vi "Update Histogram Window Menu Checks.vi"(8 "Error In":errorcluster, 9 "menu reference":refnum<k9>, 11 "XYGraph in":refnum<vi>) -> (0 "Error Out":errorcluster)   [LabVIEW 2019, in "Histogram Window.lvlib"]
uses:
  Histogram Window.lvlib
  Graphs/XY Graph/XY Graph Add-Ons.lvlib
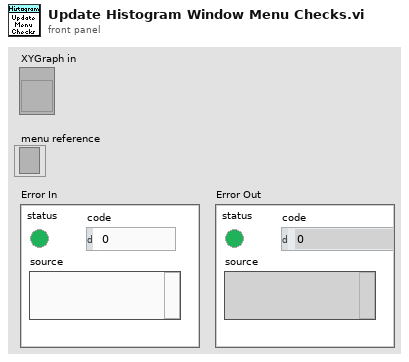
[diagram p1: front panel]
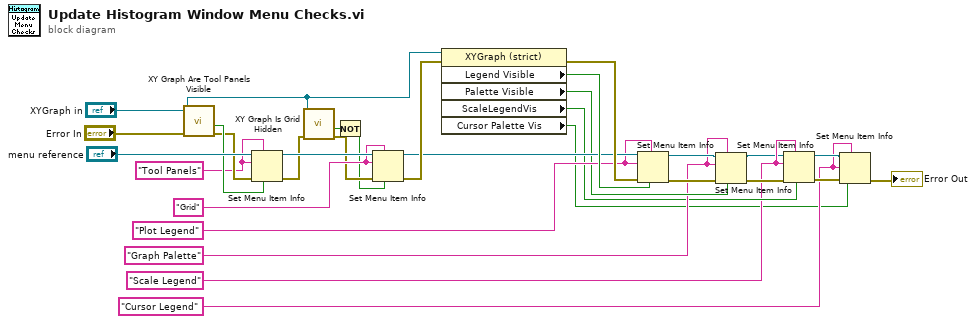
[diagram p0: block diagram]
diagram:
  w24 = "Grid" ("item name")
  w8 = "Cursor Legend" ("item name")
  w12 = "Scale Legend" ("item name")
  w15 = "Graph Palette" ("item name")
  w19 = "Plot Legend" ("item name")
  w27 = "Tool Panels" ("item name")
  n1 = call "XY Graph Are Tool Panels Visible.vi"("Error In"="Error In", "XY Graph Ref"="XYGraph in") -> ("Error Out"=w28:errorcluster, "Any Panel Visible?"=w29:bool)  [unwired: 7 in, 1 out]
  n2 = Set Menu Item Info(6:w29, 7:w27, 8:w28, 10:w27, 11:"menu reference") -> (0:w5:errorcluster, 3:w25:refnum<k9>)  [unwired: 2 in]
  n3 = call "XY Graph Is Grid Hidden.vi"("Error In"=w5, "XY Graph Ref"="XYGraph in") -> ("Error Out (dup)"=w4:errorcluster, "Hidden Grid(s)"=w3:bool)  [unwired: 7 in, 1 out]
  n4 = Not(x=w3) -> (.not. x?=w2:bool)
  n5 = Set Menu Item Info(6:w2, 7:w24, 8:w4, 10:w24, 11:w25) -> (0:w23:errorcluster, 3:w20:refnum<k9>)  [unwired: 2 in]
  n6 = property class="XYGraph (strict)"(reference="XYGraph in", error in=w23) -> (error out=w21:errorcluster, "Legend Visible"=w22:bool, "Palette Visible"=w16:bool, "ScaleLegendVis"=w13:bool, "Cursor Palette Vis"=w7:bool)  [unwired: 1 out]
  n7 = Set Menu Item Info(6:w22, 7:w19, 8:w21, 10:w19, 11:w20) -> (0:w18:errorcluster, 3:w17:refnum<k9>)  [unwired: 2 in]
  n8 = Set Menu Item Info(6:w16, 7:w15, 8:w18, 10:w15, 11:w17) -> (0:w14:errorcluster, 3:w9:refnum<k9>)  [unwired: 2 in]
  n9 = Set Menu Item Info(6:w13, 7:w12, 8:w14, 10:w12, 11:w9) -> (0:w11:errorcluster, 3:w10:refnum<k9>)  [unwired: 2 in]
  n10 = Set Menu Item Info(6:w7, 7:w8, 8:w11, 10:w8, 11:w10) -> (0:→"Error Out":errorcluster)  [unwired: 2 in, 1 out]
